vi "SmartSyntax to FormatString.vi"(0 "Structure Loop in":refnum<class "Structure Loop.lvclass">, 5 "String":string, 11 "error in (no error)":errorcluster) -> (4 "Structure Loop out":refnum<class "Structure Loop.lvclass">, 6 "Scan Syntax Format":T1, 15 "error out":errorcluster)   [LabVIEW 2016, in "Structure Loop.lvclass"]
uses:
  Structure Loop.lvclass
  common/function utils/Scan Syntax Format.ctl
  functionsbase/functionbase.lvclass
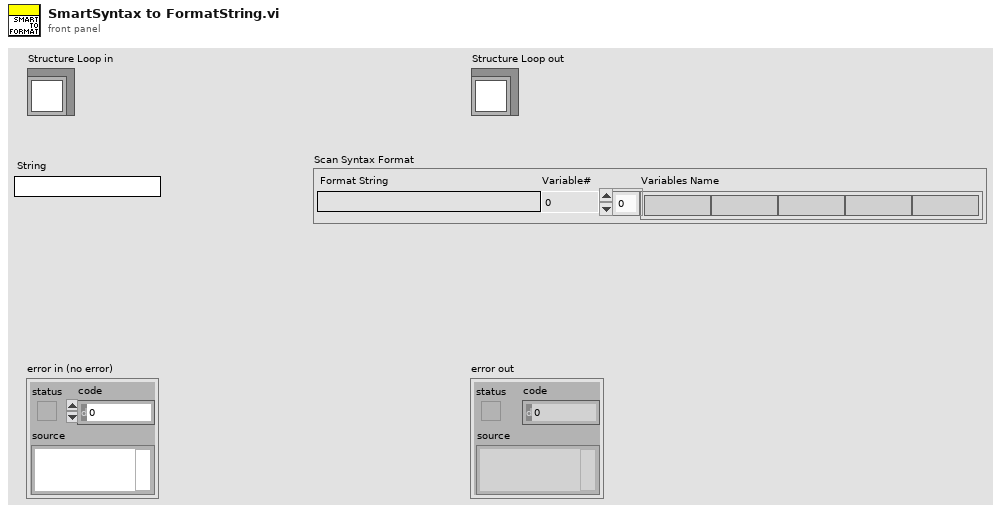
[diagram p1: front panel]
types:
  T1 = typedef "Scan Syntax Format.ctl" = cluster{"Format String":string, "Variable#":i32, "Variables Name":string[]}
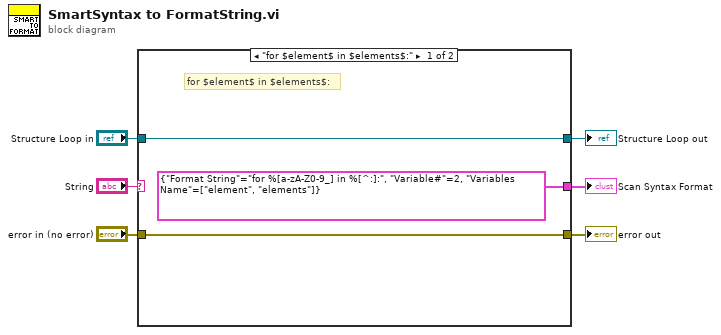
[diagram p0: block diagram]
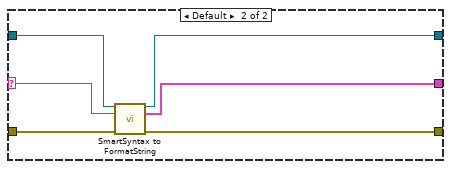
[diagram p2: hidden frame]
diagram:
  n1 = case shown="\"for $element$ in $elements$:\"" "String" {
    selector: "String" -> [_ w13]
    tunnel: "Structure Loop in" -> [w9 w15]
    tunnel: [w9 w14] -> w5
    tunnel: [T1 {"Format String"="for %[a-zA-Z0-9_] in %[^:]:", "Variable#"=2, "Variables Name"=["element", "elements"]} ("Scan Syntax Format") w12] -> w3
    tunnel: "error in (no error)" -> [w8 w11]
    tunnel: [w8 w10] -> w1
    frame "for $element$ in $elements$:" {
      # "for $element$ in $elements$:"
    }
    frame Default {
      n2 = call-parent "SmartSyntax to FormatString.vi"("functionbase in"=w15, "String"=w13, "error in (no error)"=w11) -> ("functionbase out"=w14:refnum<class "Structure Loop.lvclass">, "Scan Syntax Format"=w12:T1, "error out"=w10:errorcluster)  [unwired: 10 in]
    }
  }
  "error out" <- w1
  "Structure Loop out" <- w5
  "Scan Syntax Format" <- w3
